vi "CRC for DM3-10A.vi"(11 "CMD":u8[](array[numeric])) -> (1 "CRCLo":u8 format="%.0x", 2 "CRCHi":u8 format="%.0x", 3 "CRC for DM3-10A":u16 format="%.0x")   [LabVIEW 2015]
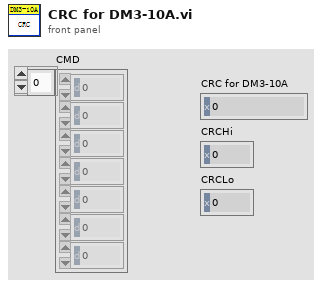
[diagram p1: front panel]
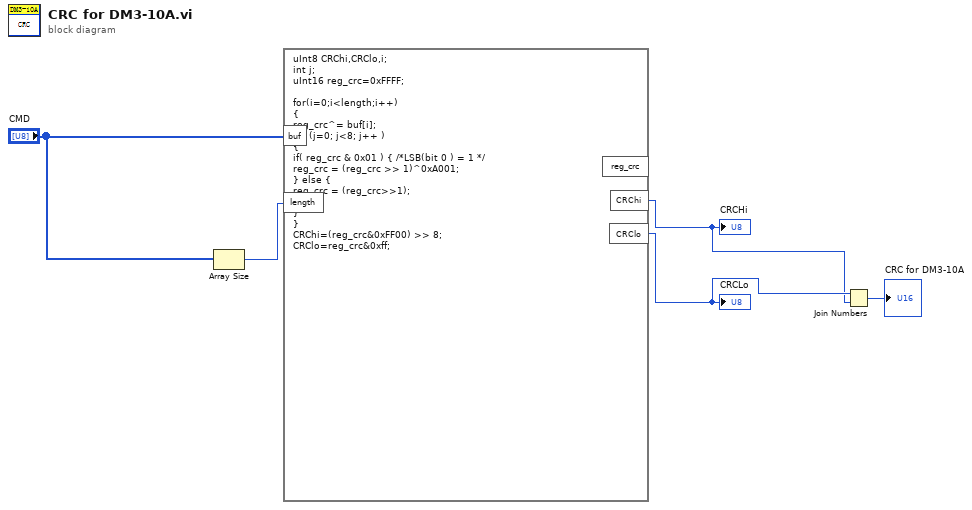
[diagram p0: block diagram]
diagram:
  n1 = Array Size(array="CMD") -> (size(s)=w5:i32)
  n2 = formula code="uInt8 CRChi,CRClo,i;\nint j; \nuInt16 reg_crc=0xFFFF; \n \nfor(i=0;i<length;i++) \n{ \nreg_crc^= buf[i]; \nfor (j=0; j<8; j++ ) \n{ \nif( reg_crc & 0x01 ) { /*LSB(bit 0 ) = 1 */ \nreg_crc = (reg_crc >> 1)^0xA001; \n} else { \nreg_crc = (reg_crc>>1); \n} \n} \n} \nCRChi=(reg_crc&0xFF00) >> 8;\nCRClo=reg_crc&0xff;"("buf"="CMD", "length"=w5) -> ("CRChi"=w2:u8, "CRClo"=w3:u8)  [unwired: 1 out]
  "CRCLo" <- w3
  "CRCHi" <- w2
  n3 = Join Numbers(hi=w3, lo=w2) -> ((hi.lo)=→"CRC for DM3-10A":u16)
